vi "Asymmetry Plot - Main.vi"(10 "Response":dbl[](array[numeric]), 11 "Stimulus":dbl[](array[numeric])) -> ()   [LabVIEW 2016]
panel:
  out "XY Graph":cluster{"Stimulus":dbl[], "Response":dbl[]}(graph)
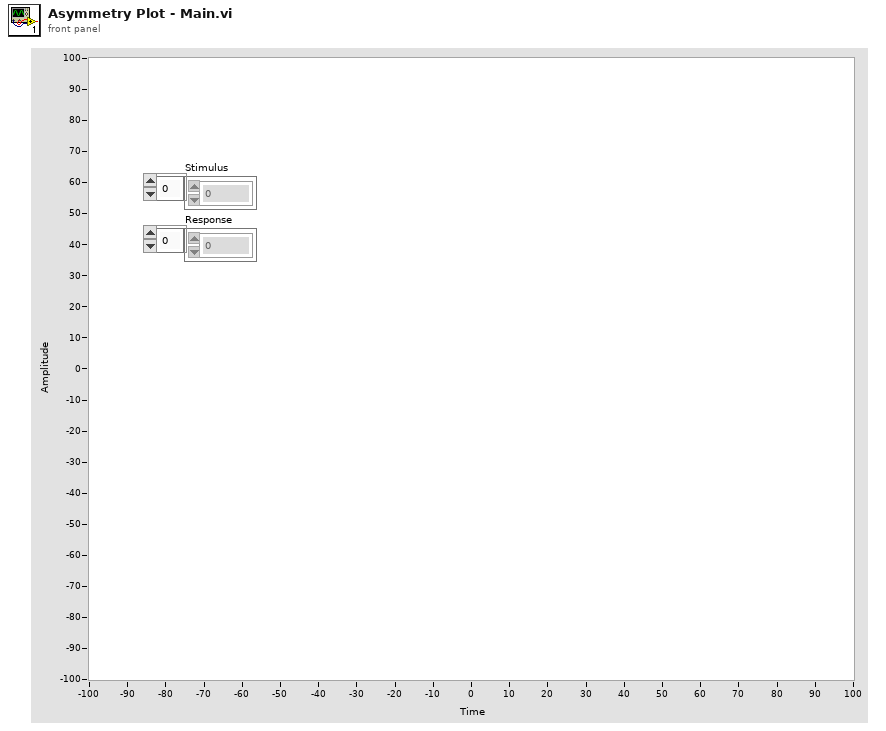
[diagram p1: front panel]
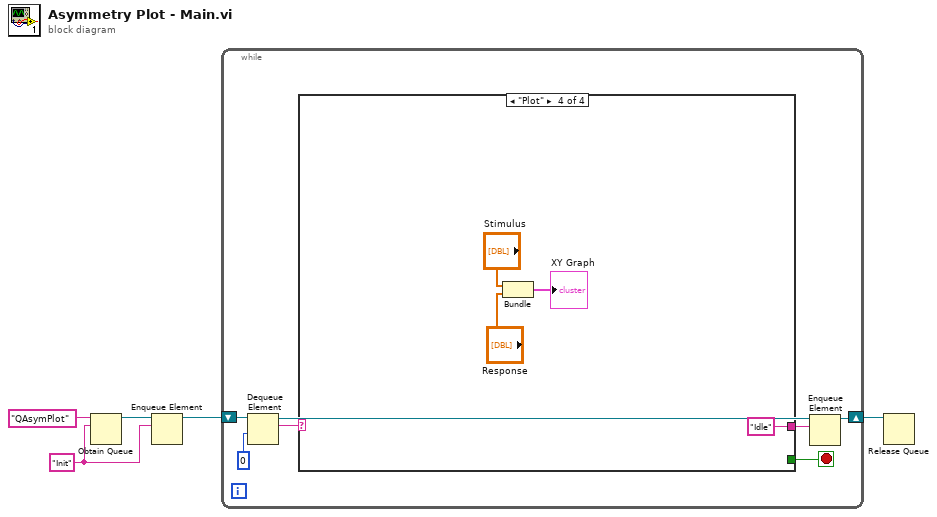
[diagram p0: block diagram]
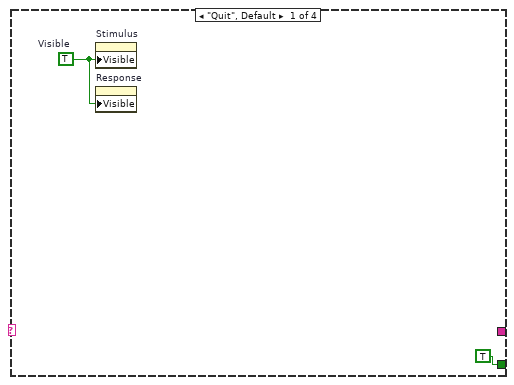
[diagram p2: hidden frame]
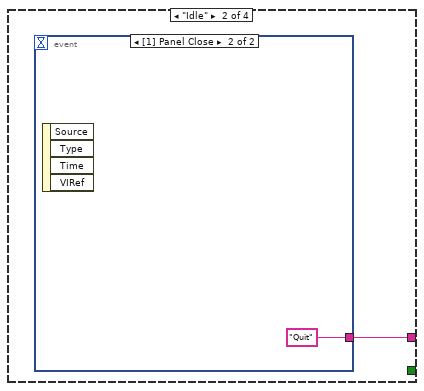
[diagram p3: hidden frame]
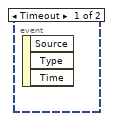
[diagram p4: hidden frame]
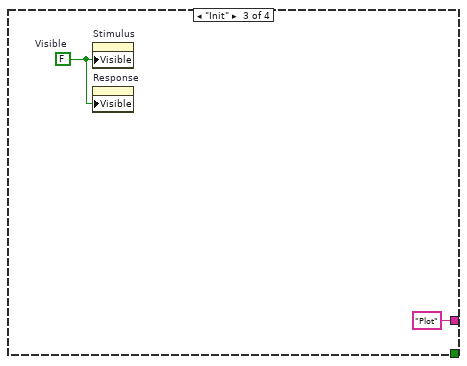
[diagram p5: hidden frame]
diagram:
  w3 = "Init" ("element")
  n1 = Obtain Queue(name (unnamed)="QAsymPlot", element data type=w3) -> (queue out=w4:refnum<queue>)  [unwired: 3 in, 2 out]
  n2 = Enqueue Element(queue=w4, element=w3) -> (queue out=w2:refnum<queue>)  [unwired: 2 in, 2 out]
  n3 = while {
    shift-right: [w10] -> w1
    shift-left: w2 -> [w12]
    stop <- w6 stop-if-true
    n4 = Dequeue Element(queue=w12, timeout in ms (-1)=0) -> (queue out=w9:refnum<queue>, element=w11:string)  [unwired: 1 in, 2 out]
    n5 = case shown="\"Plot\"" w11 {
      tunnel: [_ w15 "Plot" "Idle"] -> w8
      tunnel: [TRUE _ _ _] -> w6
      frame "Quit", Default {
        w13 = TRUE  # Visible
        n6 = property on="Stimulus" class="Arr (strict)"("Visible"=w13) -> ()  [unwired: 2 in, 2 out]
        n7 = property on="Response" class="Arr (strict)"("Visible"=w13) -> ()  [unwired: 2 in, 2 out]
      }
      frame "Idle" {
        n8 = event shown="[1] Panel Close" {
          selector: _ -> [_ _]
          dyn-events: _ -> [_ _]
          timeout: _ -> [_ _]
          tunnel: [_ "Quit"] -> w15
          event Timeout {
            n9 = event-data() -> ()  [unwired: 1 in, 3 out]
          }
          event Panel Close {
            n10 = event-data() -> ()  [unwired: 1 in, 4 out]
          }
        }
      }
      frame "Init" {
        w18 = FALSE  # Visible
        n11 = property on="Stimulus" class="Arr (strict)"("Visible"=w18) -> ()  [unwired: 2 in, 2 out]
        n12 = property on="Response" class="Arr (strict)"("Visible"=w18) -> ()  [unwired: 2 in, 2 out]
      }
      frame "Plot" {
        n13 = Bundle("Stimulus"="Stimulus", "Response"="Response") -> (→"XY Graph":cluster{"Stimulus":dbl[], "Response":dbl[]})  [unwired: 1 in]
      }
    }
    n14 = Enqueue Element(queue=w9, element=w8) -> (queue out=w10:refnum<queue>)  [unwired: 2 in, 2 out]
  }
  n15 = Release Queue(queue=w1) -> ()  [unwired: 2 in, 3 out]
